vi "IR-Read_Test.vi"() -> ()   [LabVIEW 2019]
panel:
  out "輸出紅外線值(圖)":dbl[](array[slide]) scale=0.0..3.3
  in  "Stop":bool
  out "輸出紅外線值":dbl[](array[numeric])
  in  "Reset":bool
  out "Error Out":errorcluster
  in  "Error In":errorcluster
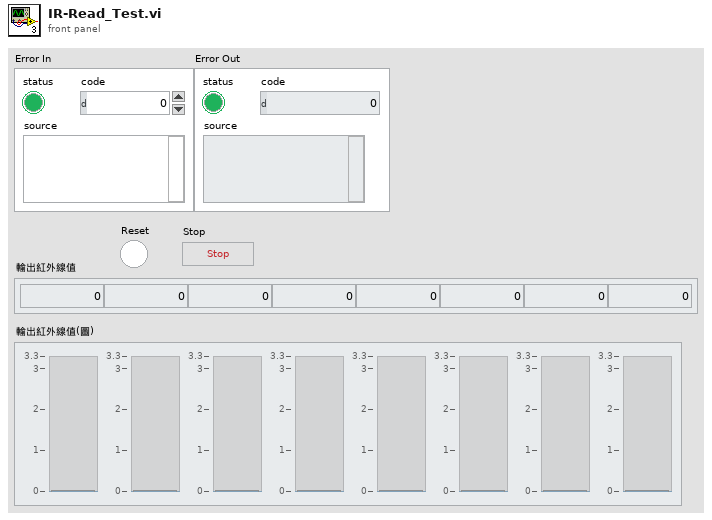
[diagram p1: front panel]
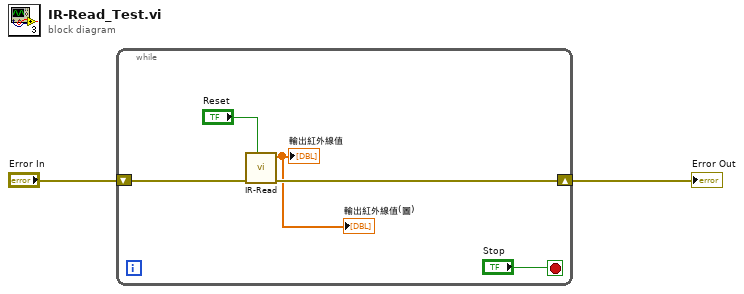
[diagram p0: block diagram]
diagram:
  n1 = while {
    shift-right: [w6] -> w1
    shift-left: "Error In" -> [w7]
    stop <- "Stop" stop-if-true
    n2 = call "IR-Read.vi"("Reset"="Reset", "Error In"=w7) -> ("Error Out"=w6:errorcluster, "輸出紅外線值"=→"輸出紅外線值" →"輸出紅外線值(圖)":dbl[])  [unwired: 8 in]
  }
  "Error Out" <- w1
